vi "RSZVL_SetRefLevel.vi"(8 "error in (no error)":errorcluster {"code" format="%.0x"}, 10 "Reference Level (-20.0)":dbl=-20.0, 11 "VISA resource name in":refnum<visa-resource-name>) -> (0 "error out":errorcluster, 3 "VISA resource name out":refnum<visa-resource-name>)   [LabVIEW 2015]
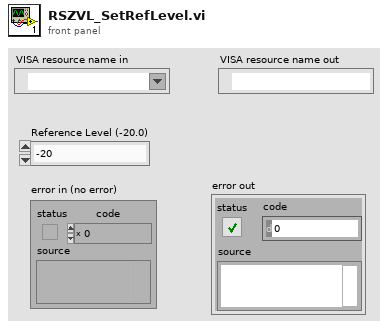
[diagram p1: front panel]
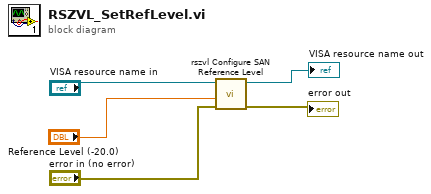
[diagram p0: block diagram]
diagram:
  n1 = call <instrlib>:"rszvl Configure SAN Reference Level.vi"("error in (no error)"="error in (no error)", "Reference Level (-20.0)"="Reference Level (-20.0)", "VISA resource name"="VISA resource name in") -> ("error out"=→"error out":errorcluster, "VISA resource name out"=→"VISA resource name out":refnum<visa-resource-name>)  [unwired: 7 in]
